vi "Path to Short Name (Unicode).vi"(8 "error in":errorcluster, 11 "Path":refnum<class "UTF-8 Path.lvclass">) -> (0 "error out":errorcluster, 3 "LabVIEW Path":path)   [LabVIEW 2020, in "G-Unicode.lvlib"]
doc: "Converts the UTF-8 path to the corresponding 8.3 short name path. Note that the path must exist on disk.\n\nThe short name path is ASCII encoded, and can be used by LabVIEW's standard file I/O functions. This allows accessing unicode paths within LabVIEW.\n\n<b>Windows only.</b> Linux and macOS will return a UTF-8 encoded path."
uses:
  G-Unicode.lvlib
  Types/UTF-8 Path/UTF-8 Path.lvclass
  Types/UTF-8 Path/UTF-8 Path.lvclass/UTF-8 Path.ctl
  Types/UTF-8 String/UTF-8 String.lvclass/UTF-8 String.ctl
  26bf929a-9a2b-411e-920d-bd75197c0103.vi
  f844562b-b612-4fa1-b092-3cf87b2107aa.vi
  Private/Conversion/Path as Path.vi
  Private/Conversion/Polymorphic VIs/Path as Path (UTF-8 Path).vi
  Private/Conversion/Text as Encoded String.vi
  Private/Conversion/Polymorphic VIs/Text as Encoded String (UTF-8 Path).vi
  Types/UTF-8 String/Write Encoded UTF-8 String.vi
  Private/Memory/Copy String.vi
  Private/Library/Result To Error.vi
  Types/UTF-8 Path/Read Encoded UTF-8 Path.vi
  Private/Memory/Copy String.vi/4d47babd-4a2d-4eb7-b91b-7e707d692665.vi
  Private/Library/gu_free.vi
  <vilib>/Utility/error.llb/Error Cluster From Error Code.vi
  Types/UTF-8 String/UTF-8 String.lvclass
  Private/Conversion/Polymorphic VIs/Text as Encoded Path (UTF-8 Path).vi
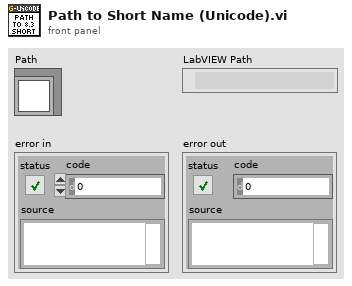
[diagram p1: front panel]
types:
  T1 = typedef "G-Unicode.lvlib/Encoded UTF-8 String.ctl" = string
  T2 = typedef "G-Unicode.lvlib/Encoded UTF-8 Path.ctl" = path
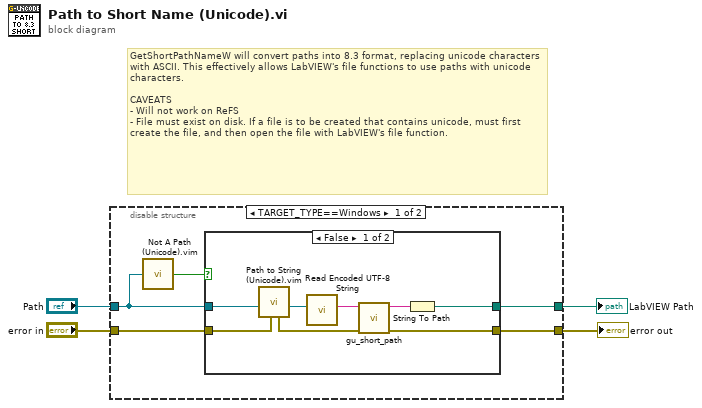
[diagram p0: block diagram]
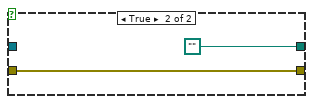
[diagram p2: hidden frame]
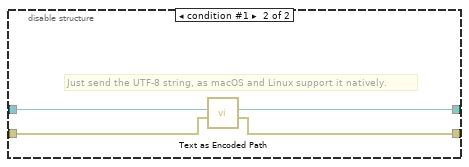
[diagram p3: hidden frame]
diagram:
  # "GetShortPathNameW will convert paths into 8.3 format, replacing unicode characters with ASCII. This effectively allows LabVIEW's file functions to use paths with unicode characters.\n\nCAVEATS\n- Will not work on ReFS\n- File must exist on disk. If a file is to be created that contains unicode, must first create the file, and then open the file with LabVIEW's file function."
  n1 = disable-structure shown="TARGET_TYPE==Windows" {
    disable-tunnel: [w8 w22] -> w1
    disable-tunnel: "Path" -> [w6 w23]
    disable-tunnel: "error in" -> [w7 w21]
    disable-tunnel: [w9 w20] -> w2
    frame condition #0 (active) {
      n2 = call "Not A Path (Unicode).vim"("Path"=w6) -> ("Path?"=w5:bool)
      n3 = case shown="False" w5 {
        tunnel: [w15 w18] -> w9
        tunnel: [w16 path ""] -> w8
        tunnel: w7 -> [w17 w18]
        tunnel: w6 -> [w14 _]
        frame False {
          n4 = call "Path to String (Unicode).vim"("error in"=w17, "Path"=w14) -> ("String"=w13:refnum<class "UTF-8 String.lvclass">, "error out"=w10:errorcluster)  [unwired: 8 in]
          n5 = call "Read Encoded UTF-8 String.vi"("UTF-8 String"=w13) -> ("Encoded UTF-8 String"=w12:T1)  [unwired: 10 in]
          n6 = call "gu_short_path.vi"("error in"=w10, "Path"=w12) -> ("error out"=w15:errorcluster, "Short Path"=w11:T1)  [unwired: 8 in]
          n7 = String To Path(string=w11) -> (path=w16:path)
        }
        frame True {
        }
      }
    }
    frame condition #1 {
      # "Just send the UTF-8 string, as macOS and Linux support it natively."
      n8 = call-poly "Text as Encoded Path.vi"("error in"=w21, "Text"=w23) -> ("error out"=w20:errorcluster, "Encoded Path"=w22:T2)  [unwired: 8 in]
    }
  }
  "LabVIEW Path" <- w1
  "error out" <- w2
